vi "Tell Forward Child.vi"(4 "Unified Actor Alias":string, 6 "Msg":refnum<class "Msg.lvclass">, 7 "Actor in":refnum<class "Actor.lvclass">, 9 "Msg DVR":refnum<data-value>) -> (0 "Error out":errorcluster, 5 "Actor out":refnum<class "Actor.lvclass">)   [LabVIEW 2020, in "jettl.lvlib"]
uses:
  jettl.lvlib
  Msg/Msg.lvclass
  Actor/Actor.lvclass
  Unified Actor Relation.ctl
  Teller.ctl
  Msg Contents/Msg Contents.lvclass
  Msg.ctl
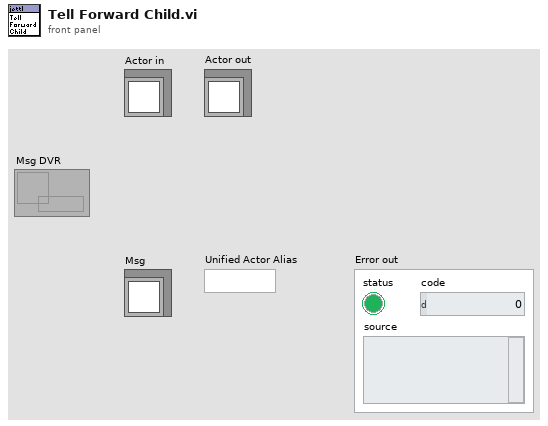
[diagram p1: front panel]
types:
  T1 = typedef "jettl.lvlib/Unified Actor.ctl" = cluster{"Msgs":T2, "Leaf":bool, "Edge Actors":refnum<class "Actor.lvclass">[], "Mid Actors":refnum<class "Actor.lvclass">[], "Core Actors":refnum<class "Actor.lvclass">[], "Root":bool, "Alias":string, "Transport":refnum<user-event>, "Address":refnum<event-registration>, "This VI":refnum<vi>}
  T2 = typedef "jettl.lvlib/Msgs.ctl" = cluster{"Inbound":T3, "Outbound":T3, "Implemented":T3, "Tell Init":T3, "Tell Init Self":T3, "Tell Init Parent":T3, "Tell Init Child":T3, "Tell Forward":T3, "Tell Forward Self":T3, "Tell Forward Parent":T3, "Tell Forward Child":T3}
  T3 = typedef "jettl.lvlib/Msg Set.ctl" = set{refnum<class "Msg.lvclass">}
  T4 = typedef "jettl.lvlib/Msg.ctl" = cluster{"Msg":refnum<class "Msg.lvclass">, "Msg Contents":refnum<class "Msg Contents.lvclass">, "Teller":T5}
  T5 = typedef "jettl.lvlib/Teller.ctl" = cluster{"Unified Actor Alias":string, "Unified Actor Relation":T6, "Absolute Time":timestamp, "Relative Time":dbl}
  T6 = typedef "jettl.lvlib/Unified Actor Relation.ctl" = enum16{"Self", "Parent", "Child"}
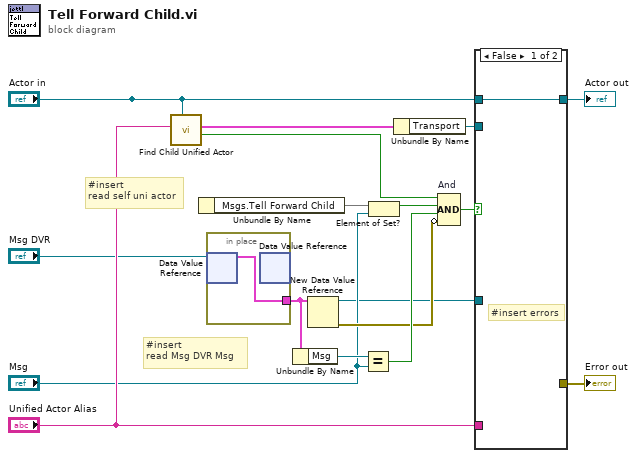
[diagram p0: block diagram]
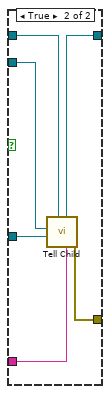
[diagram p2: hidden frame]
diagram:
  # "#insert\nread self uni actor"
  # "#insert\nread Msg DVR Msg"
  n1 = call "Find Child Unified Actor.vi"("Actor in"="Actor in", "Unified Actor Alias"="Unified Actor Alias") -> ("Found"=w4:bool, "Child Unified Actor"=w2:T1)  [unwired: 8 in]
  n2 = Unbundle By Name() -> (w8:T1, "Msgs.Tell Forward Child"=w11)
  n3 = in-place {
    in-place-border: [w19] -> w12
    n4 = in-place-dvr #1("Msg DVR") -> (w19:T4)  [unwired: 1 out]
    n5 = in-place-dvr #1() -> ()  [unwired: 1 in, 2 out]
  }
  n6 = Unbundle By Name(w12) -> ("Msg"=w13:refnum<class "Msg.lvclass">)
  n7 = New Data Value Reference(data value=w12) -> (data value reference=w5:refnum<data-value>, error out=w7:errorcluster)  [unwired: 1 in]
  n8 = Equal?(x=w13, y="Msg") -> (x = y?=w9:bool)
  n9 = Element of Set?(10:"Msg", 11:w11) -> (3:w10:bool)
  n10 = Unbundle By Name(w2) -> ("Transport"=w1:refnum<user-event>)
  n11 = Compound Arithmetic op=AND "And"(w4, w10, w9, invert w7) -> (w3:bool)
  n12 = case shown="False" w3 {
    tunnel: "Actor in" -> [w20 w26]
    tunnel: [w20 w25] -> w17
    tunnel: "Unified Actor Alias" -> [_ w23]
    tunnel: [_ w24] -> w16
    tunnel: w1 -> [_ w22]
    tunnel: w5 -> [_ w21]
    frame False {
      # "#insert errors"
    }
    frame True {
      n13 = call "Tell Child.vi"("Unified Actor Alias"=w23, "Actor in"=w26, "Msg DVR"=w21, "Transport"=w22) -> ("Error out"=w24:errorcluster, "Actor out"=w25:refnum<class "Actor.lvclass">)  [unwired: 6 in]
    }
  }
  "Error out" <- w16
  "Actor out" <- w17
